vi "Set Value.vi"(8 "error in (no error)":errorcluster, 10 "Value":i32[](array[numeric]), 11 "MulColLBTable.lvclass":refnum<class "MulColLBTable.lvclass">) -> (0 "error out":errorcluster, 3 "MulColLBTable.lvclass 2":refnum<class "MulColLBTable.lvclass">)   [LabVIEW 2020, in "MulColLBTable.lvclass"]
uses:
  MulColLBTable.lvclass
  MulColLBTable.lvclass/MulColLBTable.ctl
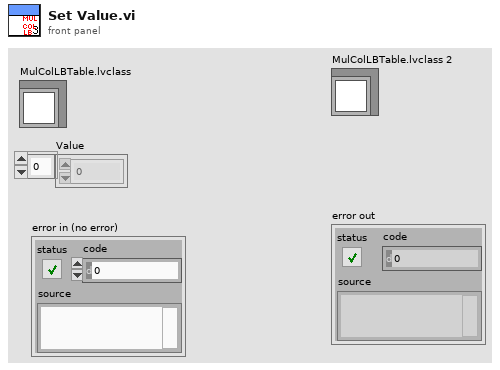
[diagram p1: front panel]
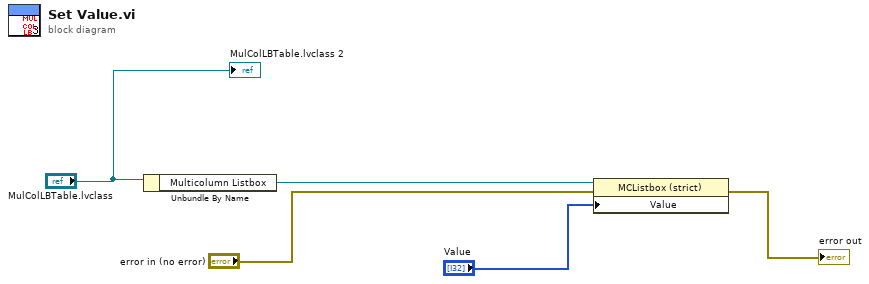
[diagram p0: block diagram]
diagram:
  n1 = Unbundle By Name("MulColLBTable.lvclass") -> ("Multicolumn Listbox"=w2:refnum<vi>)
  n2 = property class="MCListbox (strict)"(reference=w2, error in="error in (no error)", "Value"="Value") -> (error out=→"error out":errorcluster)  [unwired: 1 out]
  "MulColLBTable.lvclass 2" <- "MulColLBTable.lvclass"
